vi "debugMain.vi"(0 "Analog Input":sgl[](array[slide])=[0.0, 0.0, 0.0, 0.0, 0.0, 0.0, 0.0, 0.0] scale=0.0..5.0, 1 "Relay":cluster{"Forward":bool[], "Reverse":bool[]}={"Forward"=[FALSE, FALSE, FALSE, FALSE, FALSE, FALSE, FALSE, FALSE], "Reverse"=[FALSE, FALSE, FALSE, FALSE, FALSE, FALSE, FALSE, FALSE]}, 5 "PWM":cluster{u8, u8}[](array[slide])=[{128, 128}, {128, 128}, {128, 128}, {128, 128}, {128, 128}, {128, 128}, {128, 128}, {128, 128}, {128, 128}, {128, 128}] scale=1.0..255.0, 7 "GPIO State":bool[](array[boolean])=[FALSE, FALSE, FALSE, FALSE, FALSE, FALSE, FALSE, FALSE, FALSE, FALSE, FALSE, FALSE, FALSE, FALSE, FALSE, FALSE], 9 "Solenoids":bool[](array[boolean])=[FALSE, FALSE, FALSE, FALSE, FALSE, FALSE, FALSE, FALSE], 11 "Sensors":cluster{"Left Encoder":dbl, "Right Encoder":dbl}, 12 "GPIO Output Enable":bool[](array[boolean])=[FALSE, FALSE, FALSE, FALSE, FALSE, FALSE, FALSE, FALSE, FALSE, FALSE, FALSE, FALSE, FALSE, FALSE], 13 "Checkmarks LED array":bool[][](array[boolean])) -> (14 "Checkmarks Output LED array":bool[][](array[boolean]))   [LabVIEW 2011]
panel:
  out "CurrentStatusArray Output":bool[][](array[boolean])
  in  "CurrentStatusArray":bool[][](array[boolean])
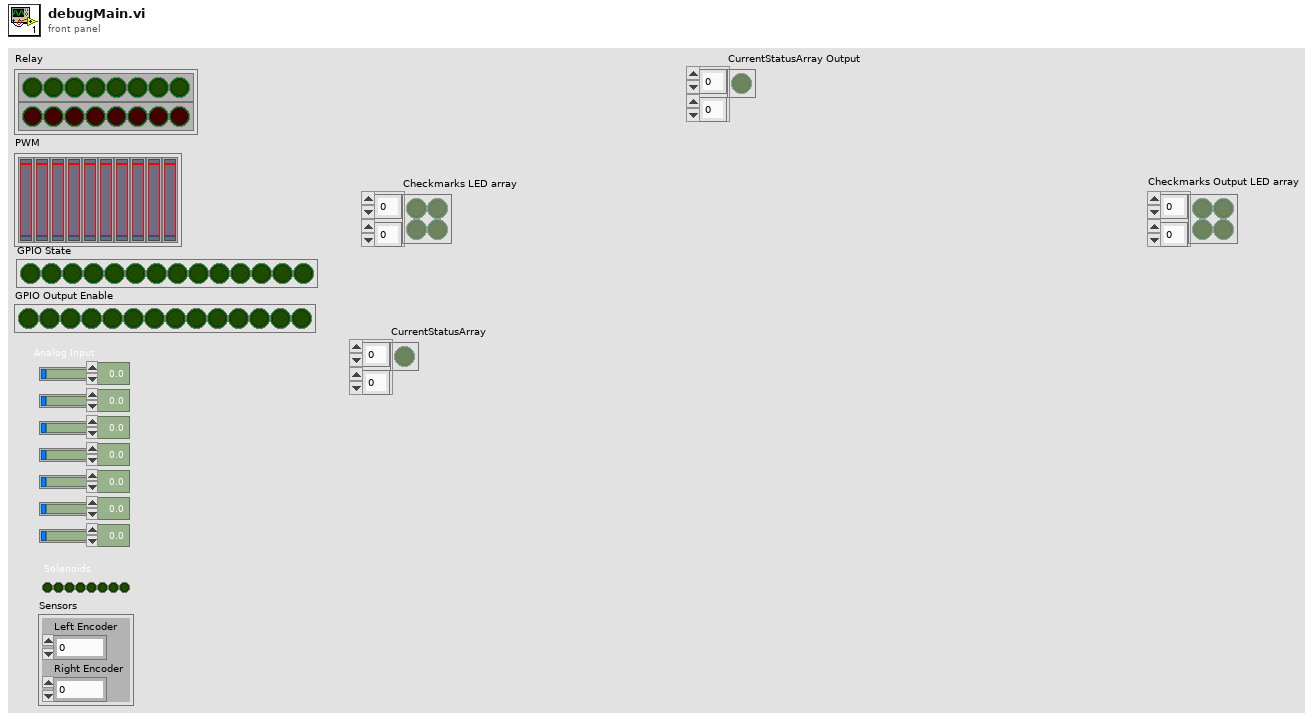
[diagram p1: front panel]
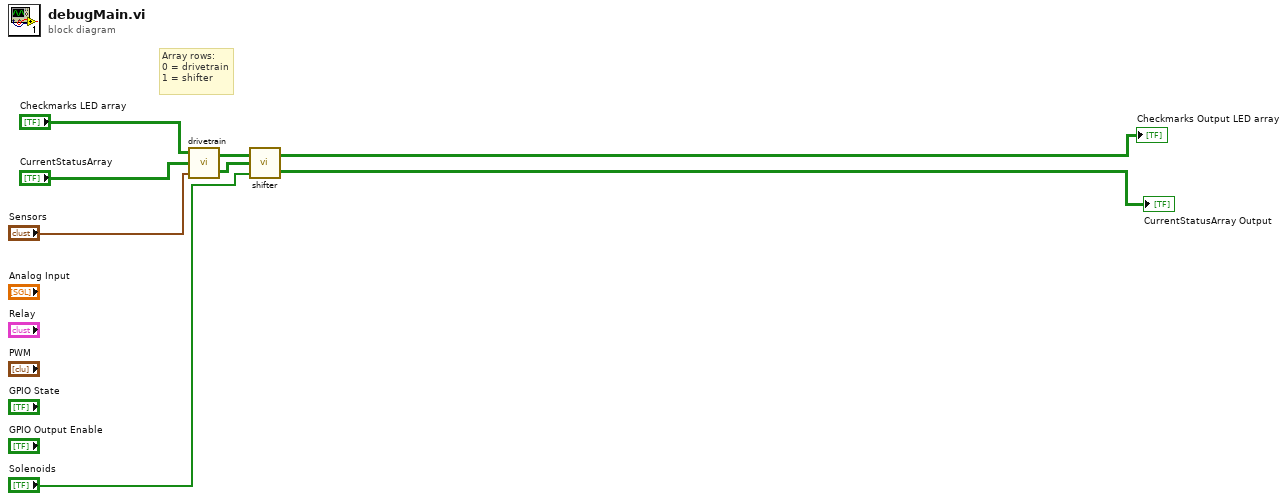
[diagram p0: block diagram]
diagram:
  # "Array rows:\n0 = drivetrain\n1 = shifter"
  n1 = call "drivetrain.vi"("Sensors"="Sensors", "CurrentStatusArray"="CurrentStatusArray", "Checkmarks Array"="Checkmarks LED array") -> ("CurrentStatusArray Output"=w4:bool[][], "Checkmarks Array Output"=w5:bool[][])
  n2 = call "shifter.vi"("Solenoids"="Solenoids", "CurrentStatusArray"=w4, "Checkmarks LED array"=w5) -> ("outputCurrentStatusArray"=→"CurrentStatusArray Output":bool[][], "outputCheckmarksArray"=→"Checkmarks Output LED array":bool[][])
